vi "Example Combined.vi"() -> ()   [LabVIEW 2015]
uses:
  <vilib>/numeric/Random Number (Range) DBL.vi
  LV QHull/QHull.lvlib
panel:
  out "error out":errorcluster
  out "XY Graph":cluster{cluster{"number":dbl, "number":dbl}[]}[](graph)
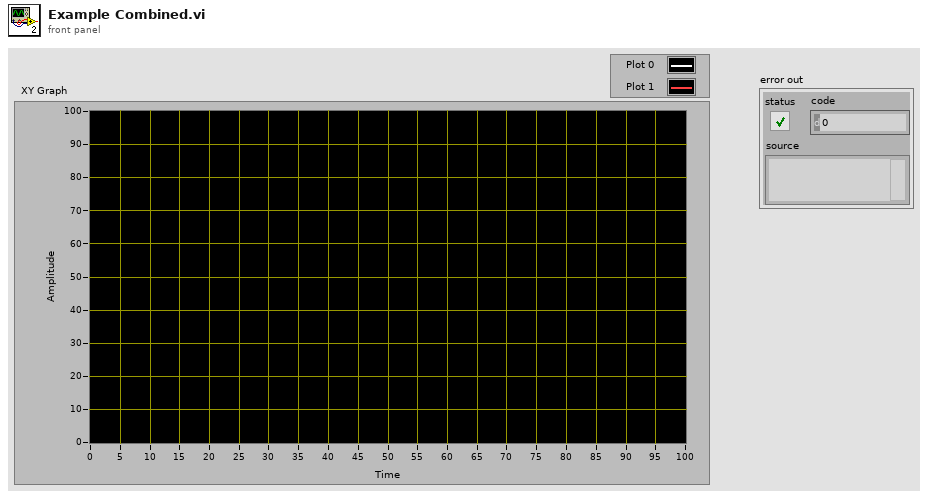
[diagram p1: front panel]
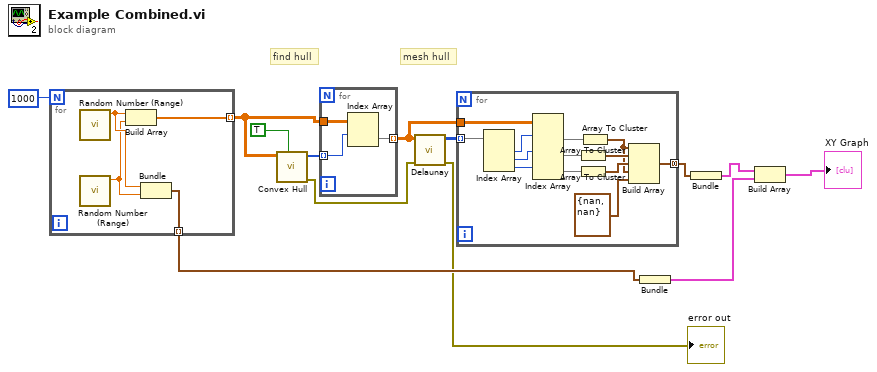
[diagram p0: block diagram]
diagram:
  # "mesh hull"
  # "find hull"
  n1 = for {
    N: 1000 -> [_]
    tunnel: [w17] -> w12 mode=indexing
    tunnel: [w14] -> w4 mode=indexing
    n2 = call-poly <vilib>:"Random Number (Range).vi"() -> ("number"=w16:dbl)  [unwired: 11 in]
    n3 = call-poly <vilib>:"Random Number (Range).vi"() -> ("number"=w15:dbl)  [unwired: 11 in]
    n4 = Build Array(w16, w15) -> (w17:dbl[])
    n5 = Bundle("number"=w16, "number"=w15) -> (w14:cluster{"number":dbl, "number":dbl})  [unwired: 1 in]
  }
  n6 = call "Convex Hull.vi"("Sort CW in 2D"=TRUE, "points"=w12) -> ("error out"=w2:errorcluster, "Simplex Indices"=w11:i32[])  [unwired: 6 in, 2 out]
  n7 = for {
    tunnel: w12 -> [w20]
    tunnel: w11 -> [w19] mode=indexing
    tunnel: [w18] -> w8 mode=indexing
    n8 = Index Array(array=w20, index (row)=w19) -> (element=w18:dbl[])  [unwired: 1 in]
  }
  n9 = call "Delaunay.vi"("error in (no error)"=w2, "points"=w8) -> ("error out"=→"error out":errorcluster, "simplices"=w10:i32[][])  [unwired: 8 in]
  n10 = for {
    tunnel: w10 -> [w32] mode=indexing
    tunnel: w8 -> [w33]
    tunnel: [w25] -> w7 mode=concatenating
    n11 = Index Array(array=w32) -> (element #1=w31:i32, element #2=w30:i32, element #3=w29:i32)  [unwired: 3 in]
    n12 = Index Array(array=w33, index (row) #1=w31, index (row) #2=w30, index (row) #3=w29) -> (element #1=w24:dbl[], element #2=w28:dbl[], element #3=w27:dbl[])  [unwired: 3 in]
    n13 = Array To Cluster(array=w28) -> (cluster=w22:cluster{"[0]":dbl, "[1]":dbl})
    n14 = Array To Cluster(array=w27) -> (cluster=w23:cluster{"[0]":dbl, "[1]":dbl})
    n15 = Array To Cluster(array=w24) -> (cluster=w21:cluster{"[0]":dbl, "[1]":dbl})
    n16 = Build Array(w21, w22, w23, w21, cluster{"number":dbl, "number":dbl} {"number"=nan, "number"=nan} ("element")) -> (w25:cluster{"number":dbl, "number":dbl}[])
  }
  n17 = Bundle(w4) -> (w3:cluster{cluster{"number":dbl, "number":dbl}[]})  [unwired: 1 in]
  n18 = Bundle(w7) -> (w6:cluster{cluster{"number":dbl, "number":dbl}[]})  [unwired: 1 in]
  n19 = Build Array(w6, w3) -> (→"XY Graph":cluster{cluster{"number":dbl, "number":dbl}[]}[])
